vi "MsgBalloon.vi"(8 "Error in":errorcluster caption="Error in (no error)", 9 "timeout (ms)":i32=1000, 10 "strCaption":string, 11 "strText":string) -> (0 "Error out":errorcluster)   [LabVIEW 2013]
uses:
  <userlib>/_SmartBalloon/Balloon Generic/Aesthetics.ctl
  <userlib>/_SmartBalloon/Balloon/Text Balloon.lvclass
  <userlib>/_SmartBalloon/Engine/Engine.lvclass
  <userlib>/_SmartBalloon/Balloon Generic/Balloon.lvclass
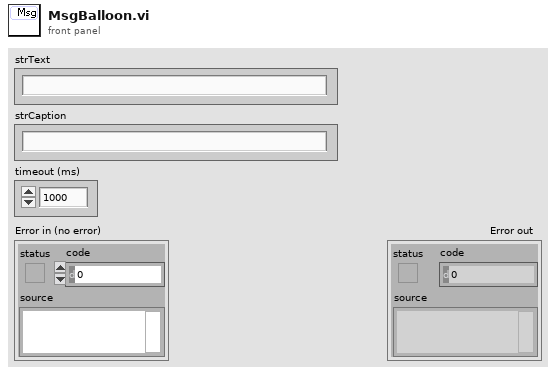
[diagram p1: front panel]
types:
  T1 = typedef "Balloon Engine.lvlib/Balloon.lvclass/Aesthetics.ctl" = cluster{"Colors":cluster{"Font Color":u32, "Panel Color":u32}, "Position":enum16{"Top", "Bottom"}, "Display Time (ms)":i32}
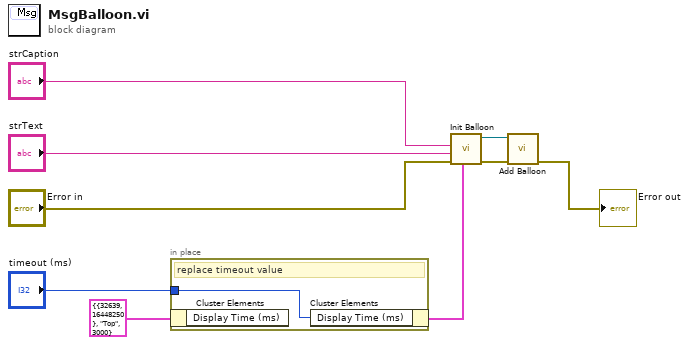
[diagram p0: block diagram]
diagram:
  n1 = in-place {
    in-place-border: "timeout (ms)" -> [w10]
    # "replace timeout value"
    n2 = in-place-cluster #1(T1 {"Colors"={"Font Color"=32639, "Panel Color"=16448250}, "Position"=enum."Top", "Display Time (ms)"=3000} ("Aesthetics")) -> ()  [unwired: 1 out]
    n3 = in-place-cluster #1("Display Time (ms)"=w10) -> (w2:T1)
  }
  n4 = call <userlib>:"Init Balloon.vi"("Aesthetics"=w2, "error in (no error)"="Error in", "Body"="strText", "Title"="strCaption") -> ("error out"=w8:errorcluster, "Balloon out"=w9:refnum<class "Text Balloon.lvclass">)  [unwired: 6 in]
  n5 = call <userlib>:"Add Balloon.vi"("error in (no error)"=w8, "Next Balloon"=w9) -> ("error out"=→"Error out":errorcluster)  [unwired: 9 in]
